vi "Get Panel Controls and VI Ref.vi"(8 "error in (no error)":errorcluster, 11 "Panel View.lvclass":refnum<class "Panel View.lvclass">) -> (0 "error out":errorcluster, 2 "Controls and VI Refnum":T1, 3 "Panel View.lvclass out":refnum<class "Panel View.lvclass">)   [LabVIEW 2015, in "Panel View.lvclass"]
uses:
  Panel View.lvclass
  Panel Manager/Type Definition/Controls and VI Refnums.ctl
  Panel View.lvclass/Panel View.ctl
  Panel Manager/Panel Manager Controller.lvclass
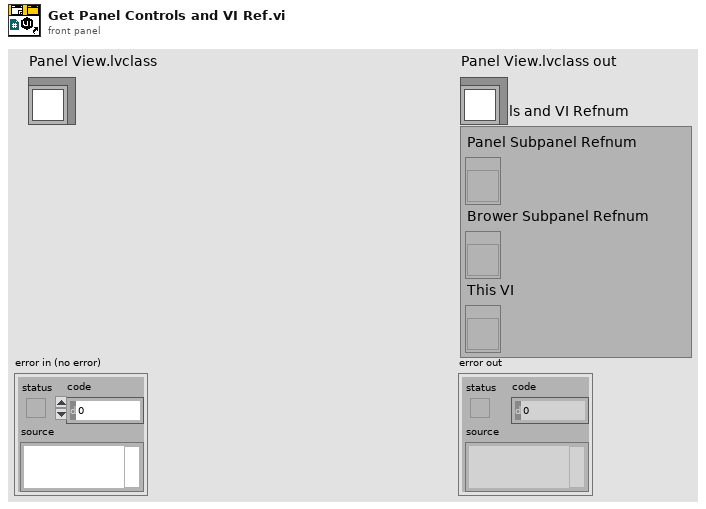
[diagram p1: front panel]
types:
  T1 = typedef "Panel Manager Controller.lvclass/Controls and VI Refnums.ctl" = cluster{"Panel Subpanel Refnum":refnum<vi>, "Brower Subpanel Refnum":refnum<vi>, "This VI":refnum<vi>}
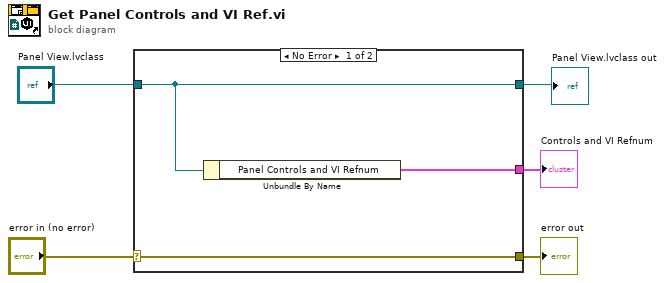
[diagram p0: block diagram]
diagram:
  n1 = case shown="No Error" "error in (no error)" {
    selector: "error in (no error)" -> [w8 w9]
    tunnel: [w8 w9] -> w4
    tunnel: [w7 w10] -> w1
    tunnel: "Panel View.lvclass" -> [w7 w10]
    tunnel: [w6 _] -> w3
    frame No Error {
      n2 = Unbundle By Name(w7) -> ("Panel Controls and VI Refnum"=w6:T1)
    }
    frame Error {
    }
  }
  "error out" <- w4
  "Controls and VI Refnum" <- w3
  "Panel View.lvclass out" <- w1
